vi "LS 340 Set Ramp.vi"(6 "Ramp on":bool, 8 "error in (no error)":errorcluster, 9 "Ramp rate, K/min":dbl=1.0, 10 "Output #":i32=1, 11 "VISA resource name":refnum<visa-resource-name>) -> (0 "error out":errorcluster, 3 "VISA Resource Name Out":refnum<visa-resource-name>)   [LabVIEW 2024]
uses:
  Simple VISA Reader/Simple VISA Reader Driver.lvclass
  GPIB/VISA  Send Receive.vi
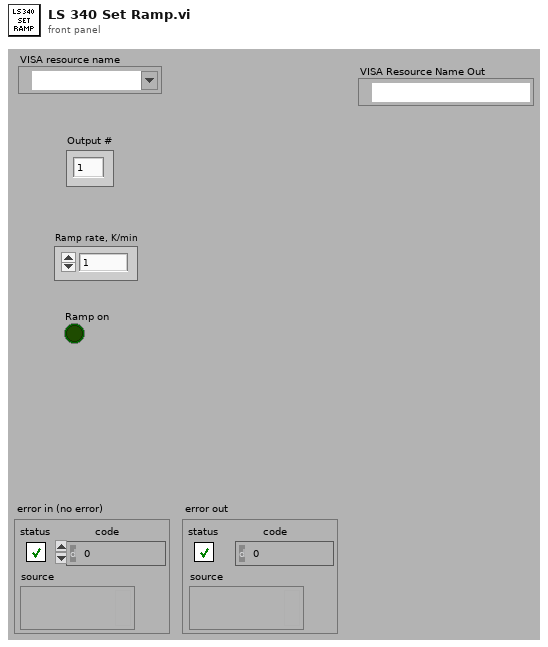
[diagram p1: front panel]
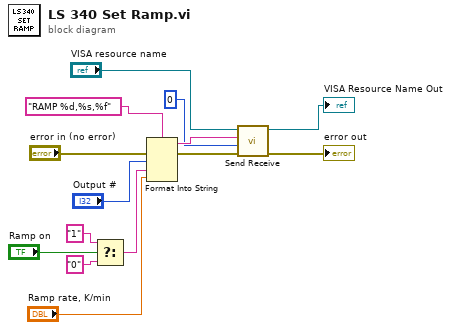
[diagram p0: block diagram]
diagram:
  n1 = Select(t="1" ("x"), s="Ramp on", f="0" ("x")) -> (s? t:f=w8:string)
  n2 = Format Into String(format string="RAMP %d,%s,%f", error in="error in (no error)", "Output #", w8, "Ramp rate, K/min") -> (resulting string=w2:string, error out=w4:errorcluster)  [unwired: 1 in]
  n3 = call-poly "Send Receive.vi"("error in (no error)"=w4, "Receive count"=0, "data string in"=w2, "VISA Resource Name"="VISA resource name") -> ("error out"=→"error out":errorcluster, "VISA Resource Name Out"=→"VISA Resource Name Out":refnum<visa-resource-name>)  [unwired: 5 in, 1 out]
